vi "FlexDDS-NG_DCP_WriteDRSS.vi"(6 "Ramp type":enum32{"Frequency", "Phase", "Amplitude"}(ring), 8 "increment step size":dbl format="%#_6f", 9 "decrement step size":dbl format="%#_6f", 10 "Channels":T1(ring)=enum."Both channels", 11 "initial instruction string":string) -> (3 "appended instruction string":string="dcp spi:DRSS=0x0\r")   [LabVIEW 2016]
panel:
  # "NOTE: Limit depends on ramp type:\nFrequency: in Hz\nAmplitude: in unit 0..1\nPhase: in degrees (0..360)"
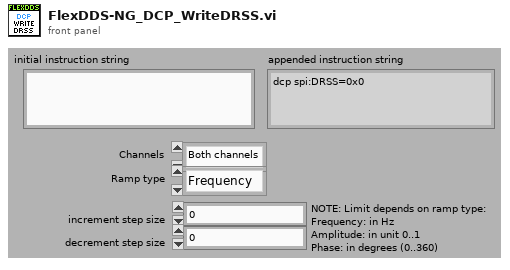
[diagram p1: front panel]
types:
  T1 = enum32{"Channel 0", "Channel 1", "Both channels"}
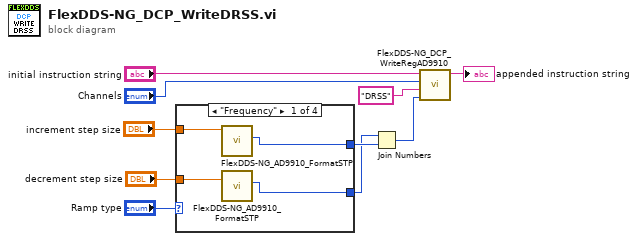
[diagram p0: block diagram]
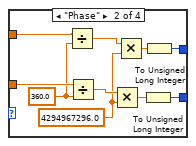
[diagram p2: hidden frame]
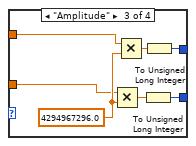
[diagram p3: hidden frame]
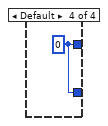
[diagram p4: hidden frame]
diagram:
  n1 = case shown="\"Frequency\"" "Ramp type" {
    tunnel: "increment step size" -> [w14 w19 w25 _]
    tunnel: "decrement step size" -> [w13 w21 w26 _]
    tunnel: [w12 w24 w31 w32] -> w1
    tunnel: [w11 w23 w30 w32] -> w2
    frame "Frequency" {
      n2 = call "FlexDDS-NG_AD9910_FormatSTP.vi"("Frequency MHz (0..400M)"=w14) -> ("frequency tuning word (FTW) out"=w11:u32)  [unwired: 7 in, 3 out]
      n3 = call "FlexDDS-NG_AD9910_FormatSTP.vi"("Frequency MHz (0..400M)"=w13) -> ("frequency tuning word (FTW) out"=w12:u32)  [unwired: 7 in, 3 out]
    }
    frame "Phase" {
      w16 = 4294967296.0 ("y")
      w18 = 360.0 ("y")
      n4 = Divide(x=w19, y=w18) -> (x/y=w17:dbl)
      n5 = Divide(x=w21, y=w18) -> (x/y=w22:dbl)
      n6 = Multiply(x=w22, y=w16) -> (x*y=w20:dbl)
      n7 = Multiply(x=w17, y=w16) -> (x*y=w15:dbl)
      n8 = To Unsigned Long Integer(number=w20) -> (unsigned 32bit integer=w24:u32)
      n9 = To Unsigned Long Integer(number=w15) -> (unsigned 32bit integer=w23:u32)
    }
    frame "Amplitude" {
      w28 = 4294967296.0 ("y")
      n10 = Multiply(x=w26, y=w28) -> (x*y=w29:dbl)
      n11 = Multiply(x=w25, y=w28) -> (x*y=w27:dbl)
      n12 = To Unsigned Long Integer(number=w29) -> (unsigned 32bit integer=w31:u32)
      n13 = To Unsigned Long Integer(number=w27) -> (unsigned 32bit integer=w30:u32)
    }
    frame Default {
      w32 = u32 0 ("frequency tuning word (FTW) out")
    }
  }
  n14 = Join Numbers(hi=w1, lo=w2) -> ((hi.lo)=w3:u64)
  n15 = call "FlexDDS-NG_DCP_WriteRegAD9910.vi"("register content"=w3, "AD9910 register name"="DRSS" ("format string"), "Channels"="Channels", "initial instruction string"="initial instruction string") -> ("appended instruction string"=→"appended instruction string":string)  [unwired: 7 in]
